vi "17_DC Motor_PID_test_2.vi"() -> ()   [LabVIEW 2018]
uses:
  <userlib>/KNR OS 4.0 LabVIEW Toolkit/Type Definition/DC Motor Port.ctl
  <userlib>/KNR OS 4.0 LabVIEW Toolkit/Type Definition/Resource.ctl
panel:
  out "Desire Velosity (cm/sec) 2":dbl
  in  "Desire Velosity (cm/sec)":dbl=30.0 format="%#_13g"
  in  "switch":bool
  in  "Port":T1=4 items=["DS1"=4, "DS2"=5, "DS3"=6, "DS4"=7]
  out "Velocity (cm/sec) Chart":dbl(graph)
  out "Speed (+-100%)":dbl
  in  "Kd":dbl(slide)=0.1 scale=0.0..0.4
  in  "Ki":dbl(slide)=0.05 scale=0.0..0.2
  in  "Kp":dbl(slide)=0.2 scale=0.0..1.0
  in  "stop":bool
  in  "Enable Motor":bool
  out "Velocity (cm/sec)":dbl
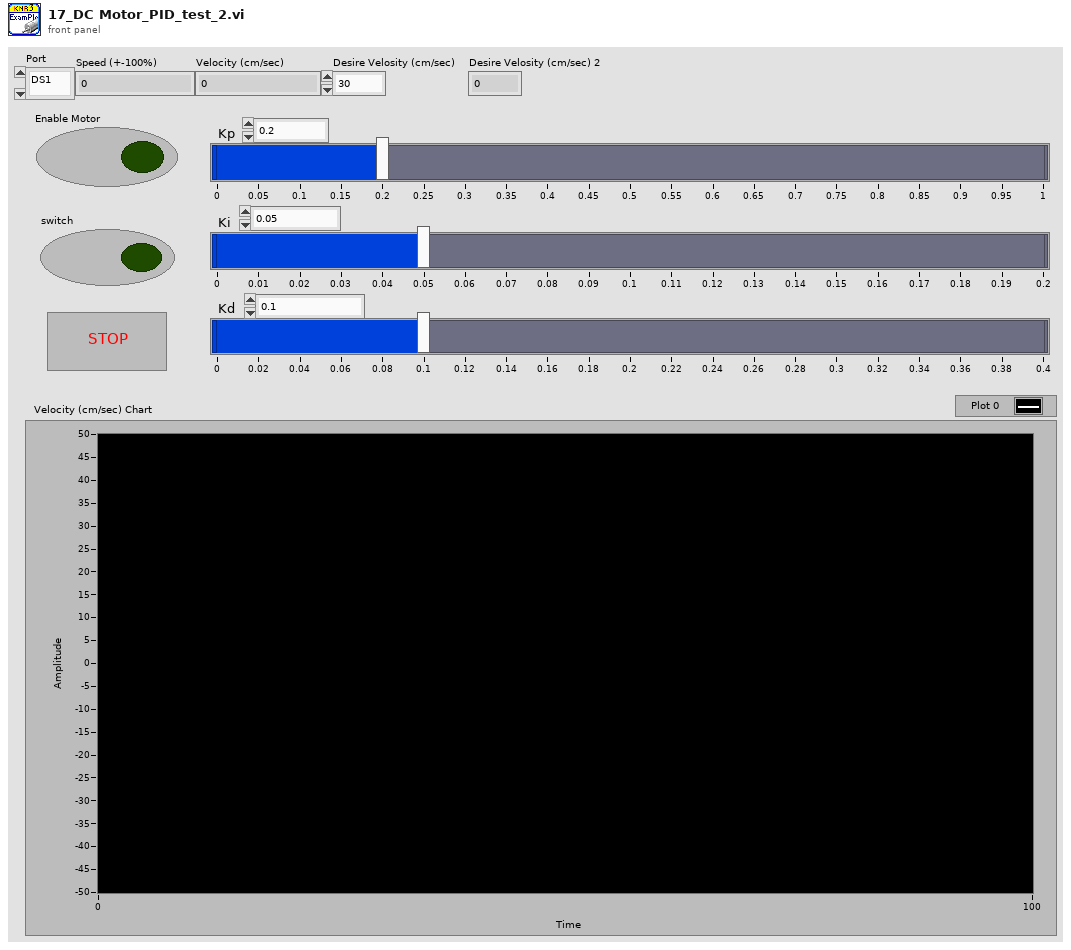
[diagram p1: front panel]
types:
  T1 = typedef "DC Motor Port.ctl" = u16
  T2 = typedef "Resource.ctl" = enum16{"KNRm_DDRC", "KNRm_DDDD", "KNRm_DDDR", "KNRm_DDDC", "KNR", "KNRm_neww"}
  T3 = typedef "KNR3 Reference.ctl" = cluster{"FPGA Session":refnum<class "FPGA Interface Base.lvclass">, "Resource":T2}
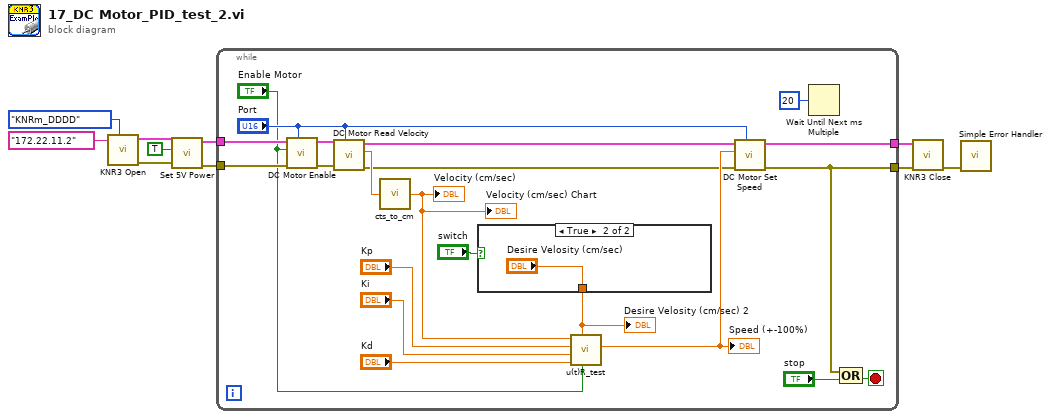
[diagram p0: block diagram]
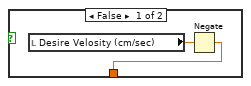
[diagram p2: hidden frame]
diagram:
  n1 = call <userlib>:"KNR3 Open.vi"("Resource"=Resource."KNRm_DDDD", "IP"="172.22.11.2") -> ("error out"=w4:errorcluster, "KNR out"=w6:T3)  [unwired: 8 in]
  n2 = call <userlib>:"Set 5V Power.vi"("error in (no error)"=w4, "5V Power(T)"=TRUE ("5V Power"), "KNR in"=w6) -> ("error out"=w8:errorcluster, "KNR out"=w9:T3)  [unwired: 7 in]
  n3 = while {
    tunnel: w9 -> [w31]
    tunnel: w8 -> [w30]
    tunnel: [w22] -> w2
    tunnel: [w21] -> w1
    stop <- w28 stop-if-true
    n4 = call <userlib>:"DC Motor Enable.vi"("Port (DS1)"="Port", "error in (no error)"=w30, "Enable Motor(F)"="Enable Motor", "KNR in"=w31) -> ("error out"=w25:errorcluster, "KNR out"=w26:T3)  [unwired: 6 in]
    n5 = call <userlib>:"DC Motor Read Velocity.vi"("Port (DS1)"="Port", "error in (no error)"=w25, "KNR in"=w26) -> ("error out"=w11:errorcluster, "Velocity (cts/sec)"=w24:dbl, "KNR out"=w12:T3)  [unwired: 6 in]
    n6 = call "cts_to_cm.vi"("cts"=w24) -> ("cm"=w16:dbl)
    "Velocity (cm/sec)" <- w16
    "Velocity (cm/sec) Chart" <- w16
    n7 = case shown="True" "switch" {
      tunnel: [w32 "Desire Velosity (cm/sec)"] -> w14
      frame False {
        n8 = local read "Desire Velosity (cm/sec)"() -> (w33:dbl)
        n9 = Negate(x=w33) -> (-x=w32:dbl)
      }
      frame True {
      }
    }
    "Desire Velosity (cm/sec) 2" <- w14
    n10 = call "u(t)R_test.vi"("enable"="Enable Motor", "Desire Velosity"=w14, "Kd"="Kd", "Ki"="Ki", "Kp"="Kp", "Velocity"=w16) -> ("u(t)"=w17:dbl)  [unwired: 5 in]
    "Speed (+-100%)" <- w17
    n11 = call <userlib>:"DC Motor Set Speed.vi"("Port (DS1)"="Port", "error in (no error)"=w11, "Speed (+-100%)"=w17, "KNR in"=w12) -> ("error out"=w21:errorcluster, "KNR out"=w22:T3)  [unwired: 6 in]
    n12 = Wait Until Next ms Multiple(millisecond multiple=u32 20) -> ()  [unwired: 1 out]
    n13 = Compound Arithmetic op=OR(w21, "stop") -> (w28:bool)
  }
  n14 = call <userlib>:"KNR3 Close.vi"("error in (no error)"=w1, "KNR in"=w2) -> ("error out"=w7:errorcluster)  [unwired: 9 in]
  n15 = call <vilib>:"Simple Error Handler.vi"("error in (no error)"=w7) -> ()  [unwired: 4 in, 5 out]
